vi "ATS9350_NPT_on-FPGA_FFT_Float.vi"() -> ()   [LabVIEW 2018]
panel:
  out "XY Graph":cluster{dbl[], sgl[]}(graph)
  in  "stop":bool
  # "Connect proper signal to channel A before starting acquisition\n(e.g. 1Vpp 1kHz sine wave)"
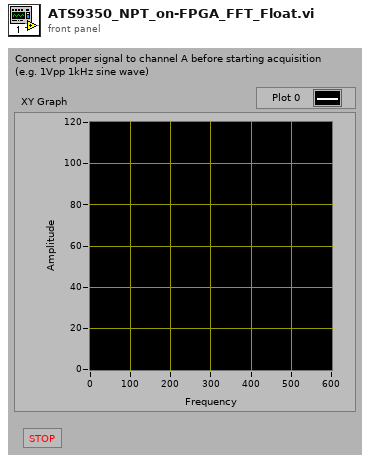
[diagram p1: front panel]
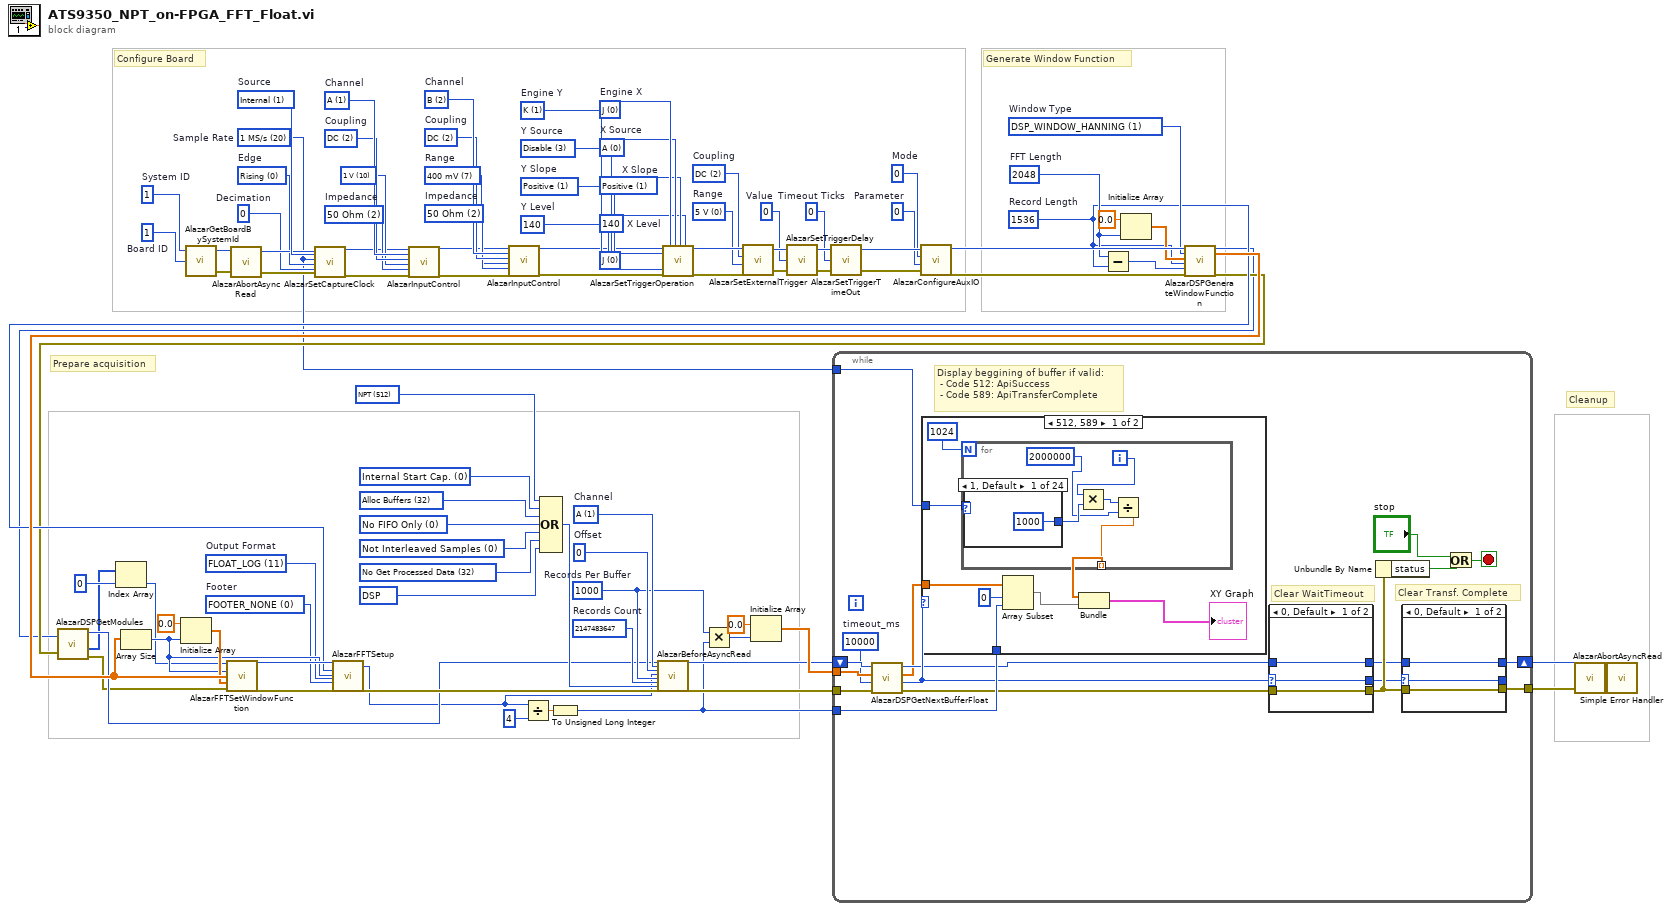
[diagram p0: block diagram]
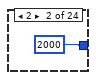
[diagram p2: hidden frame]
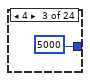
[diagram p3: hidden frame]
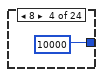
[diagram p4: hidden frame]
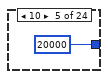
[diagram p5: hidden frame]
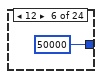
[diagram p6: hidden frame]
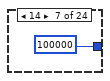
[diagram p7: hidden frame]
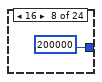
[diagram p8: hidden frame]
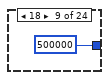
[diagram p9: hidden frame]
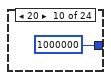
[diagram p10: hidden frame]
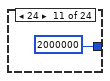
[diagram p11: hidden frame]
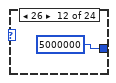
[diagram p12: hidden frame]
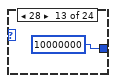
[diagram p13: hidden frame]
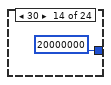
[diagram p14: hidden frame]
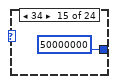
[diagram p15: hidden frame]
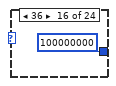
[diagram p16: hidden frame]
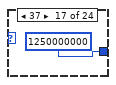
[diagram p17: hidden frame]
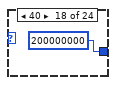
[diagram p18: hidden frame]
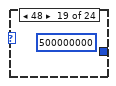
[diagram p19: hidden frame]
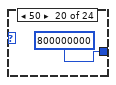
[diagram p20: hidden frame]
diagram:
  w68 = u32 10 items=["20 mV"=1, "40 mV"=2, "50 mV"=3, "80 mV"=4, "100 mV"=5, "200 mV"=6, "400 mV"=7, "500 mV"=8, "800 mV"=9, "1 V"=10, "1.25 V"=33, "2 V"=11, "4 V"=12, "5 V"=13, "8 V"=14, "10 V"=15, "20 V"=16] ("Range")
  w14 = u32 11 items=["FLOAT_AMP2"=10, "FLOAT_LOG"=11]  # Output Format
  w13 = u32 0 items=["FOOTER_NONE", "FOOTER_NPT"]  # Footer
  w28 = u32 2048  # FFT Length
  w26 = u32 1 items=["DSP_WINDOW_NONE", "DSP_WINDOW_HANNING", "DSP_WINDOW_HAMMING", "DSP_WINDOW_BLACKMAN", "DSP_WINDOW_BLACKMAN_HARRIS", "DSP_WINDOW_BARTLETT"]  # Window Type
  w16 = u32 1536  # Record Length
  w32 = u32 16384 items=["DSP"=16384]
  w62 = u32 2 items=["50 Ohm"=2]  # Impedance
  w61 = u32 7 items=["400 mV"=7]  # Range
  w63 = u32 2 items=["DC"=2]  # Coupling
  w64 = u8 2 items=["A"=1, "B"=2, "C"=4, "D"=8]  # Channel
  w40 = u32 0  # Parameter
  w39 = u32 0  # Mode
  w38 = u32 0  # Timeout Ticks
  w45 = u32 0  # Value
  w49 = u32 0 items=["5 V", "1 V", "TTL"]  # Range
  w48 = u32 2 items=["AC"=1, "DC"=2]  # Coupling
  w52 = u32 140  # Y Level
  w53 = u32 1 items=["Positive"=1, "Negative"=2]  # Y Slope
  w54 = u32 3 items=["A", "B", "External", "Disable", "C", "D"]  # Y Source
  w56 = u32 140  # X Level
  w57 = u32 1 items=["Positive"=1, "Negative"=2]  # X Slope
  w58 = u32 0 items=["A", "B", "External", "Disable", "C", "D"]  # X Source
  w55 = u32 1 items=["J", "K"]  # Engine Y
  w59 = u32 0 items=["J", "K"]  # Engine X
  w60 = u32 0 items=["J", "K", "J OR K", "J AND K", "J XOR K", "J AND NOT K", "NOT J AND K"] ("Op.")
  w67 = u32 2 items=["50 Ohm"=2]  # Impedance
  w69 = u32 2 items=["DC"=2]  # Coupling
  w70 = u8 1 items=["A"=1, "B"=2, "C"=4, "D"=8]  # Channel
  w72 = u32 0  # Decimation
  w73 = u32 0 items=["Rising", "Falling"]  # Edge
  w1 = u32 20 items=["1 kS/s"=1, "2 kS/s"=2, "5 kS/s"=4, "10 kS/s"=8, "20 kS/s"=10, "50 kS/s"=12, "100 kS/s"=14, "200 kS/s"=16, "500 kS/s"=18, "1 MS/s"=20, "2 MS/s"=24, "5 MS/s"=26, "10 MS/s"=28, "20 MS/s"=30, "50 MS/s"=34, "100 MS/s"=36, "125 MS/s"=37, "200 MS/s"=40, "500 MS/s"=48, "800 MS/s"=50, "1000 MS/s"=53, "1200 MS/s"=55, "1500 MS/s"=58, "1800 MS/s"=61, "USER_DEF"=0]  # Sample Rate
  w75 = u32 1 items=["Internal"=1, "Fast External"=2, "Medium External"=3, "Slow External"=4, "External AC"=5, "External DC"=6, "External 10MHz"=7]  # Source
  w79 = u32 1  # Board ID
  w78 = u32 1  # System ID
  w87 = u32 2147483647  # Records Count
  w12 = u32 1000  # Records Per Buffer
  w88 = u32 0  # Offset
  w33 = u32 1 items=["A"=1]  # Channel
  w95 = u32 32 items=["No Get Processed Data"=32, "Get Processed Data"=8192]
  w94 = u32 0 items=["Not Interleaved Samples"=0, "Interleave Samples"=4096]
  w90 = u32 0 items=["No FIFO Only"=0, "FIFO Only"=2048]
  w93 = u32 32 items=["Alloc Buffers"=32]
  w92 = u32 0 items=["Internal Start Cap.", "External Start Cap."]
  w91 = u32 512 items=["Traditional"=0, "NPT"=512, "Continuous"=256, "Triggered Streaming"=1024]
  # "Generate Window Function"
  # "Configure Board"
  # "Cleanup"
  # "Prepare acquisition"
  n1 = call "AlazarGetBoardBySystemId.vi"("Board ID"=w79, "System ID"=w78) -> ("error out"=w76:errorcluster, "Handle"=w77:u32)  [unwired: 1 in, 1 out]
  n2 = call "AlazarAbortAsyncRead.vi"("Handle"=w77, "error in (no error)"=w76) -> ("Handle"=w74:u32, "error out"=w71:errorcluster)  [unwired: 1 out]
  n3 = call "AlazarSetCaptureClock.vi"("Handle"=w74, "Capture Clock"=w75, 2:w1, 3:w73, 4:w72, "error in (no error)"=w71) -> ("Handle"=w66:u32, "error out"=w65:errorcluster)  [unwired: 11 in, 1 out]
  n4 = call "AlazarInputControl.vi"("Handle"=w66, "Ch Input Control"=w70, 2:w69, 3:w68, 4:w67, "error in (no error)"=w65) -> ("Handle"=w34:u32, "error out"=w37:errorcluster)  [unwired: 11 in, 1 out]
  n5 = call "AlazarInputControl.vi"("Handle"=w34, "Ch Input Control"=w64, 2:w63, 3:w61, 4:w62, "error in (no error)"=w37) -> ("Handle"=w35:u32, "error out"=w36:errorcluster)  [unwired: 11 in, 1 out]
  n6 = Compound Arithmetic op=OR(w91, w92, w93, w90, w94, w95, w32) -> (w89:u32)
  n7 = call "AlazarSetTriggerOperation.vi"("Handle"=w35, "Trigger Operation"=w60, "error in (no error)"=w36, 6:w59, 7:w55, 8:w58, 9:w54, 10:w57, 11:w53, 12:w56, 13:w52) -> ("Handle"=w51:u32, "error out"=w50:errorcluster)  [unwired: 6 in, 1 out]
  n8 = call "AlazarSetExternalTrigger.vi"("error in (no error)"=w50, "Range ID"=w49, "Coupling ID"=w48, "Handle"=w51) -> ("error out"=w46:errorcluster, "Handle"=w47:u32)  [unwired: 1 out]
  n9 = call "AlazarSetTriggerDelay.vi"("error in (no error)"=w46, "Delay"=w45, "Handle"=w47) -> ("error out"=w43:errorcluster, "Handle"=w44:u32)  [unwired: 1 out]
  n10 = call "AlazarSetTriggerTimeOut.vi"("error in (no error)"=w43, "Timeout Ticks"=w38, "Handle"=w44) -> ("error out"=w41:errorcluster, "Handle"=w42:u32)  [unwired: 1 out]
  n11 = call "AlazarConfigureAuxIO.vi"("error in (no error)"=w41, "Parameter"=w40, "Mode"=w39, "Handle"=w42) -> ("error out"=w30:errorcluster, "Handle"=w31:u32)  [unwired: 1 out]
  n12 = Subtract(x=w28, y=w16) -> (x-y=w25:u32)
  n13 = Initialize Array(sgl 0.0, w28) -> (w27:sgl[])
  n14 = call "AlazarDSPGenerateWindowFunction.vi"("Handle"=w31, "Window Type"=w26, 2:w27, 3:w16, 4:w25, "error in (no error)"=w30) -> ("Handle"=w8:u32, "window"=w24:sgl[], "error out"=w9:errorcluster)  [unwired: 10 in, 1 out]
  n15 = call "AlazarDSPGetModules.vi"("Handle"=w8, "error in (no error)"=w9) -> ("Handle"=w7:u32, "DSP Modules"=w4:u32[], "error out"=w6:errorcluster)  [unwired: 1 out]
  n16 = Index Array(array=w4, index=u32 0) -> (element=w3:u32)
  n17 = Array Size(array=w24) -> (size(s)=w15:i32)
  n18 = Initialize Array(sgl 0.0, w15) -> (w22:sgl[])
  n19 = call "AlazarFFTSetWindowFunction.vi"("DSP Handle"=w3, "Samples per record"=w15, "Real window array"=w24, "Imag window array"=w22, "error in (no error)"=w6) -> ("DSP Handle"=w21:u32, "error out"=w20:errorcluster)  [unwired: 8 in, 1 out]
  n20 = call "AlazarFFTSetup.vi"("DSP Handle"=w21, "Record Length (samples)"=w16, "FFT Length (samples)"=w15, "Output Format"=w14, "Footer"=w13, "error in (no error)"=w20) -> ("Bytes Per Output Record"=w2:u32, "error out"=w19:errorcluster)  [unwired: 18 in, 2 out]
  n21 = Divide(x=w2, y=4) -> (x/y=w17:dbl)
  n22 = To Unsigned Long Integer(number=w17) -> (unsigned 32bit integer=w10:u32)
  n23 = call "AlazarBeforeAsyncRead.vi"("Handle"=w7, "Channel Select"=w33, "Transfer Offset"=w88, "Transfer Length"=w2, "Records Per Buffer"=w12, "Records Per Acquisition"=w87, "Flags"=w89, "error in (no error)"=w19) -> ("Handle"=w84:u32, "error out"=w83:errorcluster)  [unwired: 17 in, 1 out]
  n24 = Multiply(x=w12, y=w10) -> (x*y=w11:u32)
  n25 = Initialize Array(sgl 0.0, w11) -> (w85:sgl[])
  n26 = while {
    tunnel: w85 -> [w103]
    tunnel: w83 -> [w101]
    tunnel: [w106] -> w80
    shift-right: [w107] -> w81
    shift-left: w84 -> [w104]
    tunnel: w10 -> [w105]
    tunnel: w1 -> [w96]
    stop <- w110 stop-if-true
    w102 = u32 10000  # timeout_ms
    # "Display beggining of buffer if valid:\n - Code 512: ApiSuccess\n - Code 589: ApiTransferComplete"
    # "Clear Transf. Complete"
    # "Clear WaitTimeout"
    n27 = call "AlazarDSPGetNextBufferFloat.vi"("error in (no error)"=w101, "timeout_ms"=w102, "Buffer"=w103, "Handle"=w104) -> ("error out"=w100:errorcluster, "Return Code"=w99:u32, "Buffer"=w97:sgl[], "Handle"=w98:u32)
    n28 = case shown="512, 589" w99 {
      tunnel: w97 -> [w120 _]
      tunnel: w105 -> [w119 _]
      tunnel: w96 -> [w115 _]
      frame 512, 589 {
        n29 = for {
          N: u32 1024 ("Length") -> [_]
          tunnel: w115 -> [w124]
          tunnel: [w127] -> w114 mode=indexing
          i -> [w125]
          n30 = case shown="1, Default" w124 {
            tunnel: [1000 2000 5000 10000 20000 50000 100000 200000 500000 1000000 2000000 u32 5000000 ("y") u32 10000000 ("y") u32 20000000 ("y") u32 50000000 ("y") u32 100000000 ("y") u32 1250000000 ("y") u32 200000000 ("y") _ u32 800000000 ("y") u32 1000000000 ("y") u32 1200000000 ("y") u32 1500000000 ("y") u32 1800000000 ("y")] -> w123
            frame 1, Default {
            }
            frame 2 {
            }
            frame 4 {
            }
            frame 8 {
            }
            frame 10 {
            }
            frame 12 {
            }
            frame 14 {
            }
            frame 16 {
            }
            frame 18 {
            }
            frame 20 {
            }
            frame 24 {
            }
            frame 26 {
            }
            frame 28 {
            }
            frame 30 {
            }
            frame 34 {
            }
            frame 36 {
            }
            frame 37 {
            }
            frame 40 {
            }
            frame 48 {
              (unwired) u32 500000000 ("y")
            }
            frame 50 {
            }
            frame 53 {
            }
            frame 55 {
            }
            frame 58 {
            }
            frame 61 {
            }
          }
          n31 = Multiply(x=w125, y=w123) -> (x*y=w126:u32)
          n32 = Divide(x=w126, y=u32 2000000) -> (x/y=w127:dbl)
        }
        n33 = Array Subset(array=w120, index=0, length=w119) -> (w118:sgl[])
        n34 = Bundle(w114, w118) -> (→"XY Graph":cluster{dbl[], sgl[]})  [unwired: 1 in]
      }
      frame Default {
      }
    }
    n35 = case shown="0, Default" w99 {
      selector: w99 -> [w159 w161]
      tunnel: w100 -> [w158 w164]
      tunnel: [w158 w163] -> w113
      tunnel: [w160 w162] -> w112
      tunnel: w98 -> [w160 w162]
      tunnel: [w159 w161] -> w111
      frame 0, Default {
      }
      frame 579 {
        n36 = call <vilib>:"Clear Errors.vi"("error in (no error)"=w164) -> ("error out"=w163:errorcluster)  [unwired: 5 in, 1 out]
      }
    }
    n37 = Unbundle By Name(w113) -> ("status"=w108:bool)
    n38 = case shown="0, Default" w111 {
      selector: w111 -> [w152 w154]
      tunnel: w113 -> [w151 w157]
      tunnel: [w151 w156] -> w106
      tunnel: [w153 w155] -> w107
      tunnel: w112 -> [w153 w155]
      tunnel: [w152 w154] -> _
      frame 0, Default {
      }
      frame 589 {
        n39 = call <vilib>:"Clear Errors.vi"("error in (no error)"=w157) -> ("error out"=w156:errorcluster)  [unwired: 5 in, 1 out]
      }
    }
    n40 = Or(x="stop", y=w108) -> (x .or. y?=w110:bool)
  }
  n41 = call "AlazarAbortAsyncRead.vi"("Handle"=w81, "error in (no error)"=w80) -> ("error out"=w82:errorcluster)  [unwired: 2 out]
  n42 = call <vilib>:"Simple Error Handler.vi"("error in (no error)"=w82) -> ()  [unwired: 4 in, 5 out]
